vi "Arm.vi"(8 "error in (no error)":errorcluster, 10 "Arm":bool=TRUE, 11 "Mag Lab Digitizer in":refnum<class "Mag Lab Digitizer.lvclass">) -> (0 "error out":errorcluster, 3 "Mag Lab Digitizer out":refnum<class "Mag Lab Digitizer.lvclass">)   [LabVIEW 2015, in "Mag Lab Digitizer.lvclass"]
uses:
  Mag Lab Digitizer.lvclass
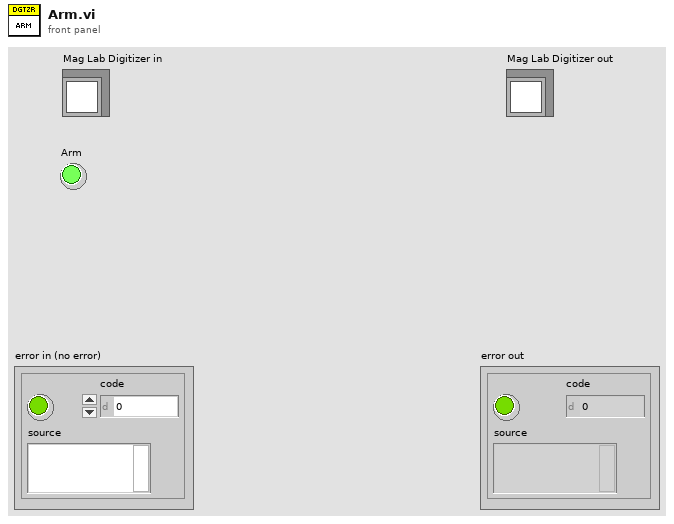
[diagram p1: front panel]
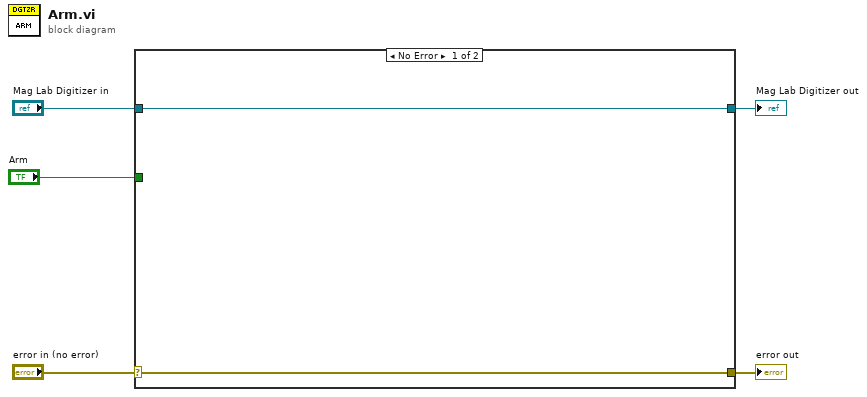
[diagram p0: block diagram]
diagram:
  n1 = case shown="No Error" "error in (no error)" {
    selector: "error in (no error)" -> [w6 w9]
    tunnel: [w6 w9] -> w4
    tunnel: [w7 w8] -> w2
    tunnel: "Mag Lab Digitizer in" -> [w7 w8]
    tunnel: "Arm" -> [_ _]
    frame No Error {
    }
    frame Error {
    }
  }
  "error out" <- w4
  "Mag Lab Digitizer out" <- w2
